vi "test_InstrumentTypeIdNotInReservation_CallCreateSessions_ReturnsErrorFor0Sessions.vi"(8 "error in":errorcluster) -> (0 "error out":errorcluster, 2 "result":string, 3 "pass":bool)   [LabVIEW 2020, in "MeasurementServerTests.lvlib"]
uses:
  MeasurementServerTests.lvlib
  da6ffb6f-c1c9-4957-84dd-e9228483c454.vi
  ffc64c76-1568-41a3-8328-b9126ac9a28d.vi
  Helpers/Fake Instrument/Fake Instrument.lvclass
  \\tsclient\C/dev/measurementlink-labview/Source/Runtime/MeasurementLink Instrument/IInstrument/IInstrument.lvclass
  Runtime/MeasurementLink Measurement Server/Helpers/Error Strings Global Internal.vi
  Runtime/MeasurementLink Session Management/Session Reservation/Create Sessions Impl.vi
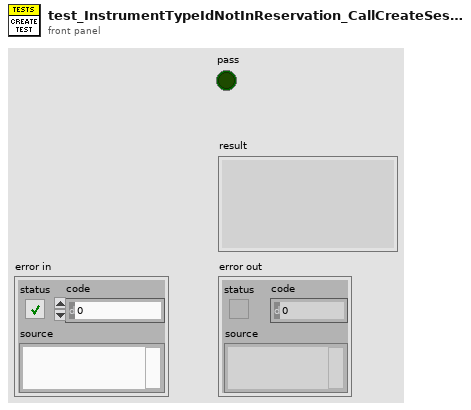
[diagram p1: front panel]
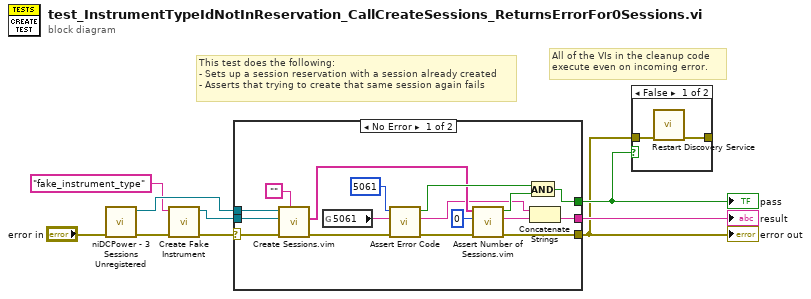
[diagram p0: block diagram]
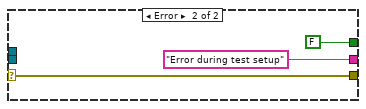
[diagram p2: hidden frame]
diagram:
  # "All of the VIs in the cleanup code\nexecute even on incoming error."
  # "This test does the following:\n- Sets up a session reservation with a session already created\n- Asserts that trying to create that same session again fails"
  n1 = call "niDCPower - 3 Sessions Unregistered.vi"("error in (no error)"="error in") -> ("error out"=w3:errorcluster, "Session Reservation out"=w2:refnum<class "Session Reservation.lvclass">)  [unwired: 9 in]
  n2 = call "Create Fake Instrument.vi"("error in"=w3, "instrument type id"="fake_instrument_type") -> ("error out"=w6:errorcluster, "fake instrument out"=w5:refnum<class "Fake Instrument.lvclass">)  [unwired: 8 in]
  n3 = case shown="No Error" w6 {
    selector: w6 -> [w24 w27]
    tunnel: [w15 w27] -> w7
    tunnel: [w14 FALSE] -> w8
    tunnel: [w12 "Error during test setup" ("f")] -> w9
    tunnel: w5 -> [w26 _]
    tunnel: w2 -> [w25 _]
    frame No Error {
      n4 = call "Create Sessions.vim"("session type"="", "error in"=w24, "instrument"=w26, "session reservation in"=w25) -> ("error out"=w23:errorcluster, "sessions"=w18:string[])  [unwired: 4 in, 2 out]
      n5 = global read "Error Strings Global Internal.vi" "5061"() -> (w19:string)
      n6 = call "Assert Error Code.vi"("error in"=w23, "expected error description"=w19, "expected error code"=5061) -> ("error out"=w16:errorcluster, "details"=w10:string, "error code match?"=w22:bool)  [unwired: 6 in]
      n7 = call "Assert Number of Sessions.vim"("error in"=w16, "expected number of sessions"=0, "sessions"=w18) -> ("error out"=w15:errorcluster, "result"=w11:string, "pass"=w13:bool)  [unwired: 6 in]
      n8 = And(x=w22, y=w13) -> (x .and. y?=w14:bool)
      n9 = Concatenate Strings(w10, w11) -> (w12:string)
    }
    frame Error {
    }
  }
  "error out" <- w7
  "pass" <- w8
  "result" <- w9
  n10 = case shown="False" w8 {
    tunnel: w7 -> [w31 _]
    tunnel: [w30 _] -> _
    frame False {
      n11 = call "Restart Discovery Service.vi"("error in"=w31) -> ("error out"=w30:errorcluster)  [unwired: 10 in]
    }
    frame True {
    }
  }
